vi "superimpose.vi"(0 "Bottom Image":T1, 5 "Top Image":T1, 7 "X":i32, 9 "Y":i32, 11 "error in (no error)":errorcluster) -> (4 "Bottom Image out":T1, 6 "Top Image out":T1, 15 "error out":errorcluster)   [LabVIEW 2017, in "Vision.lvlib"]
uses:
  Vision.lvlib
  <vilib>/vision/Image Controls.llb/IMAQ Image.ctl
  bin/Vision.dll
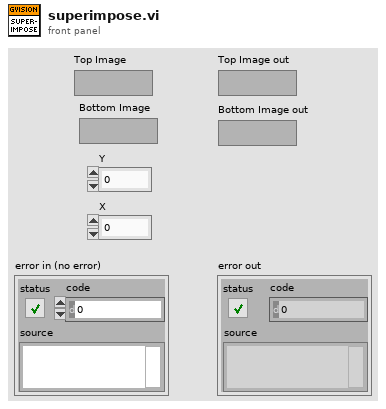
[diagram p1: front panel]
types:
  T1 = typedef "IMAQ Image.ctl" = refnum<image>
  T2 = enum32{"Map Pixel Pointer", "Unmap Pixel Pointer", "Get Pixels Infos"}
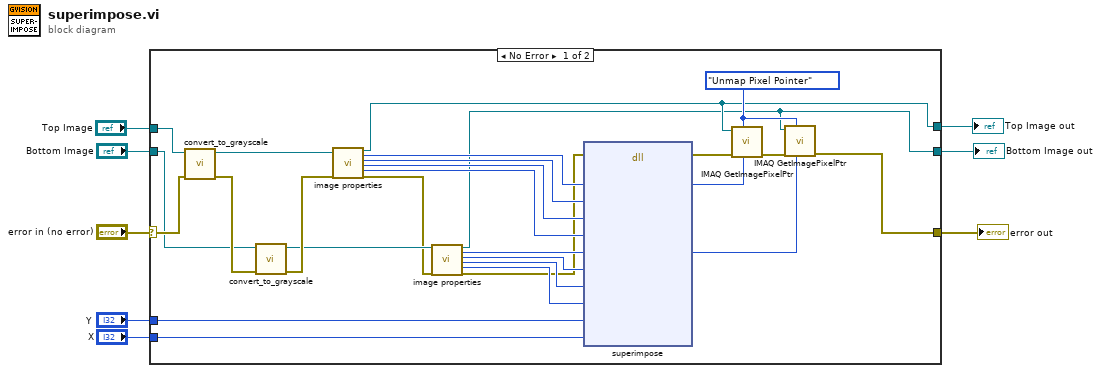
[diagram p0: block diagram]
diagram:
  n1 = case shown="No Error" "error in (no error)" {
    selector: "error in (no error)" -> [w32 w38]
    tunnel: "Bottom Image" -> [w11 w36]
    tunnel: [w13 w38] -> w6
    tunnel: [w10 w37] -> w5
    tunnel: "Y" -> [w15 _]
    tunnel: "X" -> [w14 _]
    tunnel: "Top Image" -> [w12 w37]
    tunnel: [w9 w36] -> w1
    frame No Error {
      w33 = T2."Unmap Pixel Pointer" ("Function")
      n2 = call "convert_to_grayscale.vi"("error in (no error)"=w32, "Image in"=w12) -> ("error out"=w20:errorcluster, "Image out"=w18:T1)  [unwired: 8 in]
      n3 = call "convert_to_grayscale.vi"("error in (no error)"=w20, "Image in"=w11) -> ("error out"=w19:errorcluster, "Image out"=w17:T1)  [unwired: 8 in]
      n4 = call "image properties.vi"("Image in"=w18, "error in (no error)"=w19) -> ("Image out"=w10:T1, "Pixel Pointer out"=w31:u64, "Line Width"=w30:i32, "X Resolution"=w29:i32, "Y Resolution"=w28:i32, "error out"=w16:errorcluster)  [unwired: 11 in, 1 out]
      n5 = call "image properties.vi"("Image in"=w17, "error in (no error)"=w16) -> ("Image out"=w9:T1, "Pixel Pointer out"=w27:u64, "Line Width"=w26:i32, "X Resolution"=w25:i32, "Y Resolution"=w24:i32, "error out"=w23:errorcluster)  [unwired: 11 in, 1 out]
      n6 = dll-call lib="C:/Users/Caleb/Desktop/nebraska-silicon-lab/pixel-gantry-extra/LV/bin/Vision.dll" fn="superimpose"(error in=w23, "src_imgPtr"=w31, "src_imgLineWidth"=w30, "src_imgWidth"=w29, "src_imgHeight"=w28, "dst_imgPtr"=w27, "dst_imgLineWidth"=w26, "dst_imgWidth"=w25, "dst_imgHeight"=w24, "dstTop"=w15, "dstLeft"=w14) -> (error out=w34:errorcluster, "src_imgPtr"=w22:u64, "dst_imgPtr"=w21:u64)  [unwired: 11 in, 1 out]
      n7 = call "IMAQ GetImagePixelPtr"("Pixel Pointer in"=w22, "Function"=w33, "error in (no error)"=w34, "Image"=w10) -> ("error out"=w35:errorcluster)  [unwired: 2 in, 5 out]
      n8 = call "IMAQ GetImagePixelPtr"("Pixel Pointer in"=w21, "Function"=w33, "error in (no error)"=w35, "Image"=w9) -> ("error out"=w13:errorcluster)  [unwired: 2 in, 5 out]
    }
    frame Error {
    }
  }
  "Top Image out" <- w5
  "error out" <- w6
  "Bottom Image out" <- w1
